vi "Sequence.CreateMainForLoop.vi"(8 "error in (no error)":errorcluster, 10 "IterationInfo":T1, 11 "Iterations":u32) -> (0 "error out":errorcluster, 3 "ForLoop Ref":refnum<k24>)   [LabVIEW 2015, in "Single Station Execution.lvlib"]
uses:
  Single Station Execution.lvlib
  Types/Channel.Properties.ctl
  NationalInstruments.VeriStand.RealTimeSequenceDefinitionApi
  Main.Constants.vi
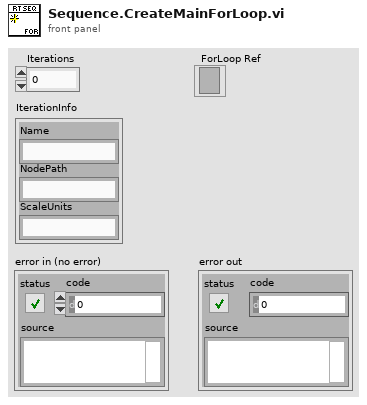
[diagram p1: front panel]
types:
  T1 = typedef "Single Station Execution.lvlib/Channel.Properties.ctl" = cluster{"Name":string, "NodePath":string, "ScaleUnits":string}
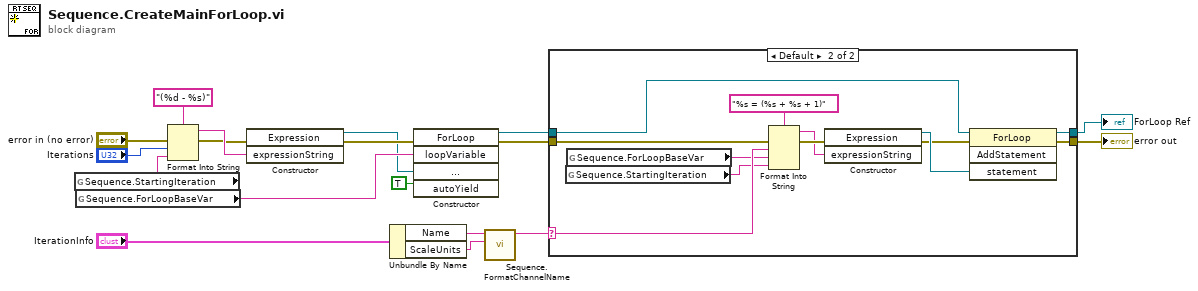
[diagram p0: block diagram]
diagram:
  n1 = global read "Main.Constants.vi" "Sequence.StartingIteration"() -> (w17:string)
  n2 = global read "Main.Constants.vi" "Sequence.ForLoopBaseVar"() -> (w18:string)
  n3 = Format Into String(format string="(%d - %s)", error in="error in (no error)", "Iterations", w17) -> (resulting string=w6:string, error out=w4:errorcluster)  [unwired: 1 in]
  n4 = constructor class="Expression"(error in=w4, "expressionString"=w6) -> (reference out=w13:refnum<k24>, error out=w14:errorcluster)  [unwired: 2 in, 2 out]
  n5 = Unbundle By Name("IterationInfo") -> ("Name"=w12:string, "ScaleUnits"=w11:string)
  n6 = constructor class="ForLoop"(error in=w14, "loopVariable"=w18, "iterations"=w13, "autoYield"=TRUE) -> (reference out=w9:refnum<k24>, error out=w10:errorcluster)  [unwired: 2 in, 4 out]
  n7 = call "Sequence.FormatChannelName.vi"("ScaleUnits"=w11, "Name"=w12) -> ("ChannelName"=w8:string)  [unwired: 9 in]
  n8 = case shown="Default" w8 {
    selector: w8 -> [_ w23]
    tunnel: [w20 w32] -> w2
    tunnel: w9 -> [w19 w31]
    tunnel: [w19 w30] -> w1
    tunnel: w10 -> [w20 w27]
    frame "" {
    }
    frame Default {
      n9 = global read "Main.Constants.vi" "Sequence.StartingIteration"() -> (w22:string)
      n10 = global read "Main.Constants.vi" "Sequence.ForLoopBaseVar"() -> (w21:string)
      n11 = Format Into String(format string="%s = (%s + %s + 1)", error in=w27, w23, w21, w22) -> (resulting string=w24:string, error out=w26:errorcluster)  [unwired: 1 in]
      n12 = constructor class="Expression"(error in=w26, "expressionString"=w24) -> (reference out=w29:refnum<k24>, error out=w28:errorcluster)  [unwired: 2 in, 2 out]
      n13 = invoke class="ForLoop" method="AddStatement"(reference=w31, error in=w28, "statement"=w29) -> (reference out=w30:refnum<k24>, error out=w32:errorcluster)  [unwired: 1 in, 2 out]
    }
  }
  "error out" <- w2
  "ForLoop Ref" <- w1
